vi "侧边栏移动.vi"(8 "错误输入（无错误）":errorcluster, 9 "留白":u32, 10 "移动方向选择":T1, 11 "控件引用输入":refnum<vi>) -> (0 "错误输出":errorcluster, 3 "引用输出":refnum<vi>)   [LabVIEW 8.6, in "窗口操作.lvlib"]
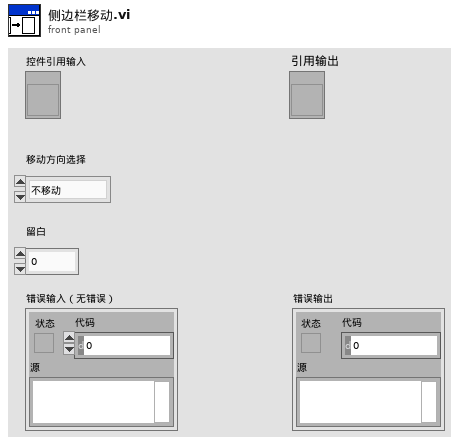
[diagram p1: front panel]
types:
  T1 = typedef "移动方向枚举.ctl" = enum16{"不移动", "向上移动", "向下移动", "向左移动", "向右移动"}
  T2 = typedef "LVBoundsTypeDef.ctl" = cluster{"Width":u32, "Height":u32}
  T3 = typedef "LVPositionTypeDef.ctl" = cluster{"Left":i32, "Top":i32}
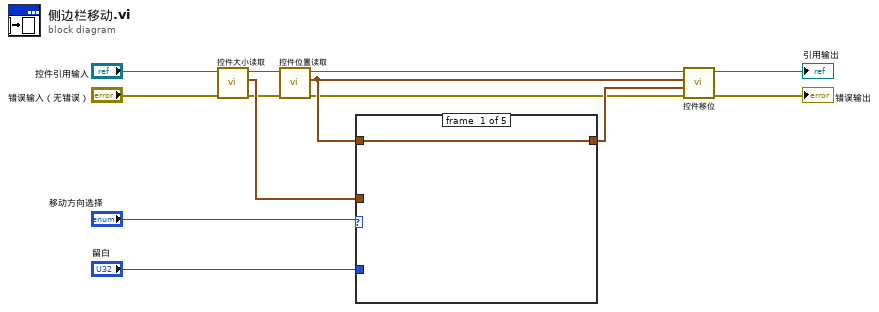
[diagram p0: block diagram]
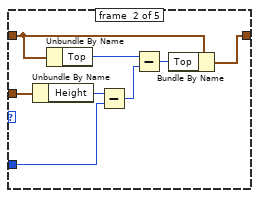
[diagram p2: hidden frame]
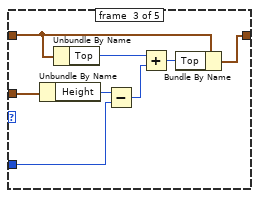
[diagram p3: hidden frame]
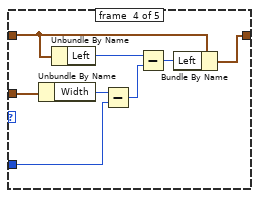
[diagram p4: hidden frame]
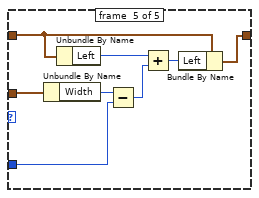
[diagram p5: hidden frame]
diagram:
  n1 = call "控件大小读取.vi"("错误输入（无错误）"="错误输入（无错误）", "控件引用输入"="控件引用输入") -> ("错误输出"=w9:errorcluster, "边界"=w12:T2, "引用输出"=w7:refnum<vi>)  [unwired: 7 in]
  n2 = call "控件位置读取.vi"("错误输入（无错误）"=w9, "控件引用输入"=w7) -> ("错误输出"=w8:errorcluster, "位置"=w11:T3)  [unwired: 7 in, 1 out]
  n3 = case shown="\"向上移动\"" "移动方向选择" {
    tunnel: w12 -> [_ w21 w25 w32 w39]
    tunnel: w11 -> [w13 w16 w22 w33 w41]
    tunnel: [w13 w14 w23 w30 w40] -> w10
    tunnel: "留白" -> [_ w15 w24 w31 w38]
    frame #0 {
    }
    frame #1 {
      n4 = Unbundle By Name(w21) -> ("Height"=w19:u32)
      n5 = Unbundle By Name(w16) -> ("Top"=w20:i32)
      n6 = Subtract(x=w19, y=w15) -> (x-y=w18:u32)
      n7 = Subtract(x=w20, y=w18) -> (x-y=w17:u32)
      n8 = Bundle By Name(cluster=w16, "Top"=w17) -> (w14:T3)
    }
    frame #2 {
      n9 = Unbundle By Name(w25) -> ("Height"=w28:u32)
      n10 = Unbundle By Name(w22) -> ("Top"=w29:i32)
      n11 = Subtract(x=w28, y=w24) -> (x-y=w27:u32)
      n12 = Add(x=w29, y=w27) -> (x+y=w26:u32)
      n13 = Bundle By Name(cluster=w22, "Top"=w26) -> (w23:T3)
    }
    frame #3 {
      n14 = Unbundle By Name(w32) -> ("Width"=w36:u32)
      n15 = Unbundle By Name(w33) -> ("Left"=w37:i32)
      n16 = Subtract(x=w36, y=w31) -> (x-y=w35:u32)
      n17 = Subtract(x=w37, y=w35) -> (x-y=w34:u32)
      n18 = Bundle By Name(cluster=w33, "Left"=w34) -> (w30:T3)
    }
    frame #4 {
      n19 = Unbundle By Name(w39) -> ("Width"=w44:u32)
      n20 = Unbundle By Name(w41) -> ("Left"=w45:i32)
      n21 = Subtract(x=w44, y=w38) -> (x-y=w43:u32)
      n22 = Add(x=w45, y=w43) -> (x+y=w42:u32)
      n23 = Bundle By Name(cluster=w41, "Left"=w42) -> (w40:T3)
    }
  }
  n24 = call "控件移位.vi"("错误输入（无错误）"=w8, "终点"=w10, "起始点"=w11, "控件引用输入"=w7) -> ("错误输出"=→"错误输出":errorcluster, "引用输出"=→"引用输出":refnum<vi>)  [unwired: 6 in]
